vi "Get Class Default Object.vi"(8 "error in (no error)":errorcluster, 10 "Class Path/Name":string, 11 "CS++Factory in":refnum<class "CS++Factory.lvclass">) -> (0 "error out":errorcluster, 2 "Class Default Object":refnum<class>, 3 "CS++Factory out":refnum<class "CS++Factory.lvclass">)   [LabVIEW 2015, in "CS++BaseClasses.lvlib" / "CS++Factory.lvclass"]
doc: "This is a dynamic dispatch VI.\n\n It is used to return an object with LabVIEW class default value. It becomed loaded from disk using <b>Class</b> as path. If the class is not found or an error is generated it ti tried to return a class default object from memory. \n\nThis helps testing classes during development and building application with statically linked classes with all dependencies.\n\nDerived classes can override this VI in order to load classes into memory as plugin, e.g. precompiled lvlibs."
uses:
  CS++Factory.lvclass
  Libraries/Utilities/CS++Utilities.lvlib
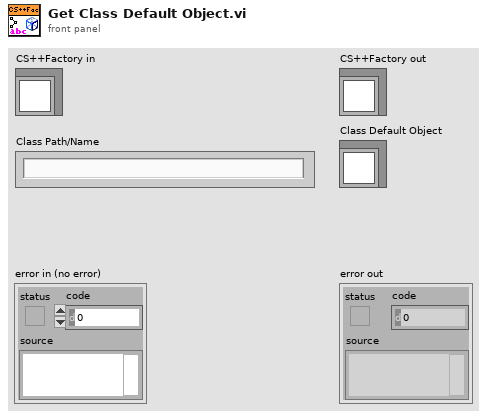
[diagram p1: front panel]
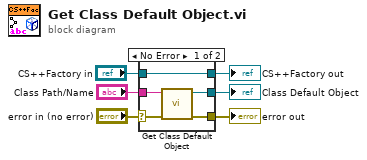
[diagram p0: block diagram]
diagram:
  n1 = case shown="No Error" "error in (no error)" {
    selector: "error in (no error)" -> [w9 w13]
    tunnel: [w8 w13] -> w5
    tunnel: [w11 w12] -> w3
    tunnel: "CS++Factory in" -> [w11 w12]
    tunnel: "Class Path/Name" -> [w10 _]
    tunnel: [w7 _] -> w1
    frame No Error {
      n2 = call "Get Class Default Object.vi"("Error In"=w9, "Class"=w10) -> ("Error Out"=w8:errorcluster, "Class Default Object"=w7:refnum<class>)  [unwired: 8 in]
    }
    frame Error {
    }
  }
  "error out" <- w5
  "CS++Factory out" <- w3
  "Class Default Object" <- w1
